vi "Control Timeout.vi"(11 "Class 2 in":refnum<class "Class 2.lvclass">) -> (3 "Class 2 out":refnum<class "Class 2.lvclass">)   [LabVIEW 2019, in "Class 2.lvclass"]
uses:
  Class 2.lvclass
  Class 2.lvclass/Class 2.ctl
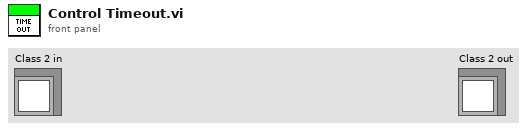
[diagram p1: front panel]
types:
  T1 = cluster{"Timeout Activado":bool, "Tiempo Timeout":u32, "Mensaje Timeout":string, "Tiempo Inicial":u32}
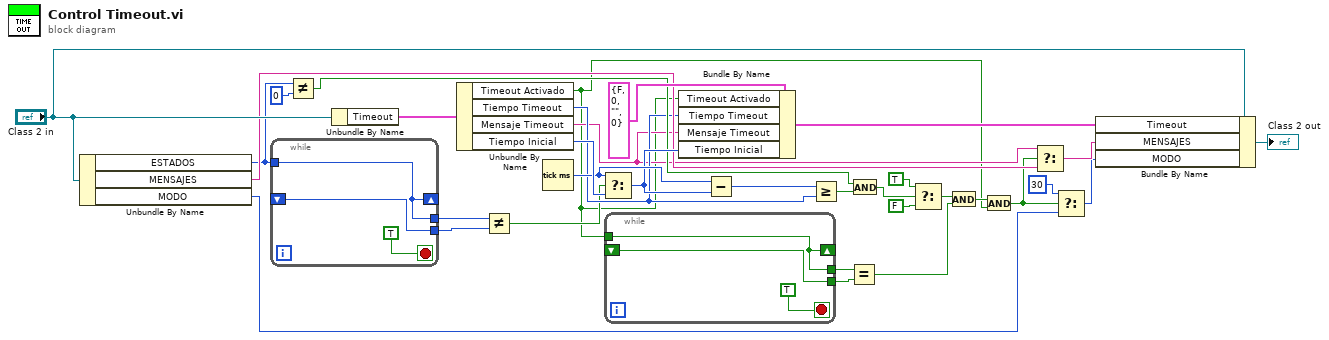
[diagram p0: block diagram]
diagram:
  n1 = Unbundle By Name("Class 2 in") -> ("ESTADOS"=w5:i16, "MENSAJES"=w17:string, "MODO"=w16:i16)
  n2 = while {
    shift-right: [w34] -> _
    shift-left: _ -> [w35]
    tunnel: w5 -> [w34]
    tunnel: [w35] -> w8
    tunnel: [w34] -> w7
    stop <- TRUE stop-if-true
  }
  n3 = Not Equal?(x=w5, y=i16 0) -> (x != y?=w24:bool)
  n4 = Unbundle By Name("Class 2 in") -> ("Timeout"=w33:T1)
  n5 = Unbundle By Name(w33) -> ("Timeout Activado"=w2:bool, "Tiempo Timeout"=w13:u32, "Mensaje Timeout"=w12:string, "Tiempo Inicial"=w31:u32)
  n6 = Not Equal?(x=w7, y=w8) -> (x != y?=w6:bool)
  n7 = Tick Count (ms)() -> (millisecond timer value=w27:u32)
  n8 = Select(t=w27, s=w6, f=w31) -> (s? t:f=w26:u32)
  n9 = while {
    shift-right: [w37] -> _
    shift-left: _ -> [w38]
    tunnel: w2 -> [w37]
    tunnel: [w38] -> w3
    tunnel: [w37] -> w4
    stop <- TRUE stop-if-true
  }
  n10 = Bundle By Name(cluster=T1 {"Timeout Activado"=FALSE, "Tiempo Timeout"=0, "Mensaje Timeout"="", "Tiempo Inicial"=0} ("Timeout"), "Timeout Activado"=w2, "Tiempo Timeout"=w13, "Mensaje Timeout"=w12, "Tiempo Inicial"=w26) -> (w28:T1)
  n11 = Subtract(x=w27, y=w26) -> (x-y=w25:u32)
  n12 = Greater Or Equal?(x=w25, y=w13) -> (x >= y?=w23:bool)
  n13 = Equal?(x=w4, y=w3) -> (x = y?=w1:bool)
  n14 = And(x=w24, y=w23) -> (x .and. y?=w21:bool)
  n15 = Select(t=TRUE, s=w21, f=FALSE) -> (s? t:f=w11:bool)
  n16 = And(x=w11, y=w1) -> (x .and. y?=w10:bool)
  n17 = And(x=w10, y=w2) -> (x .and. y?=w9:bool)
  n18 = Select(t=w12, s=w9, f=w17) -> (s? t:f=w18:string)
  n19 = Select(t=i16 30, s=w9, f=w16) -> (s? t:f=w15:i16)
  n20 = Bundle By Name(cluster="Class 2 in", "Timeout"=w28, "MENSAJES"=w18, "MODO"=w15) -> (→"Class 2 out":refnum<class "Class 2.lvclass">)
